vi "Find Edges.vi"(7 "Find Edge setting":T8={"Options"={"Search Direction"=0, "Edge Options"={"Edge Polarity"=0, "Kernel Size"=3, "Width"=3, "Minimum Edge Strength"=10.0, "Interpolation Type"=enum."Bilinear Fixed", "Data Processing Method"=enum."Average"}, "Show Search Area"=FALSE, "Show Search Lines"=FALSE, "Show Edges Found"=FALSE, "Show Result"=TRUE, "Search Area Color"=65280, "Search Lines Color"=255, "Edge Locations Color"=16776960, "Result Color"=16711680, "Overlay Group Name"=""}, "Line Fit Options"={"Number of Lines"=1, "Type"=enum."First Edge Rake", "Min. Score"=10.0, "Max. Score"=1000.0, "Orientation"=0.0, "Angle Range"=45.0, "Angle Tolerance"=1.0, "Step Size"=7, "Min. SNR (db)"=0.0, "Min. Points (%)"=25.0, "Hough Iterations"=5}} {"Options"."Search Direction" items=["Left to Right", "Right to Left", "Top to Bottom", "Bottom to Top"]; "Options"."Edge Options"."Edge Polarity" items=["All Edges", "Rising Edges", "Falling Edges"]; "Options"."Edge Options"."Minimum Edge Strength" format="%.2f"; "Options"."Edge Options"."Width" step=2; "Options"."Edge Options"."Kernel Size" step=2; "Line Fit Options"."Min. Points (%)" min=0.0 max=100.0; "Line Fit Options"."Min. SNR (db)" min=0.0; "Line Fit Options"."Max. Score" min=0.0 max=1024.0; "Line Fit Options"."Min. Score" min=0.0 max=1024.0 step=1.0}, 8 "error in (no error)":errorcluster, 9 "Matches (pixel)":T9, 10 "ROI Descriptor":T1 {"Contours"."Type" items=["No Selection", "Point", "Line", "Rectangle", "Oval", "Polygon", "Freehand Region", "Annulus", "Unused2", "Unused3", "Broken Line", "Freehand Line", "Rotated Rectangle"]}, 11 "Image":T3) -> (0 "error out":errorcluster, 1 "Straight Edges":T2(array[cluster]) {"Point2 (Real-World)"."Y" format="%.2f"; "Point2 (Real-World)"."X" format="%.2f"; "Point1 (Real-World)"."Y" format="%.2f"; "Point1 (Real-World)"."X" format="%.2f"; "Point2 (Pixels)"."Y" format="%.2f"; "Point2 (Pixels)"."X" format="%.2f"; "Point1 (Pixels)"."Y" format="%.2f"; "Point1 (Pixels)"."X" format="%.2f"}, 2 "Found Edge?":bool, 3 "Image Out":T3)   [LabVIEW 2017]
uses:
  <vilib>/vision/Measure.llb/Edge Options.ctl
  <vilib>/vision/Measure.llb/Edge Polarity.ctl
  <vilib>/vision/Measure.llb/Straight Edge Options.ctl
  <vilib>/vision/Measure.llb/Straight Edge Process.ctl
  <vilib>/vision/Image Controls.llb/IMAQ Image.ctl
  <vilib>/vision/NI_Vision_Development_Module.lvlib
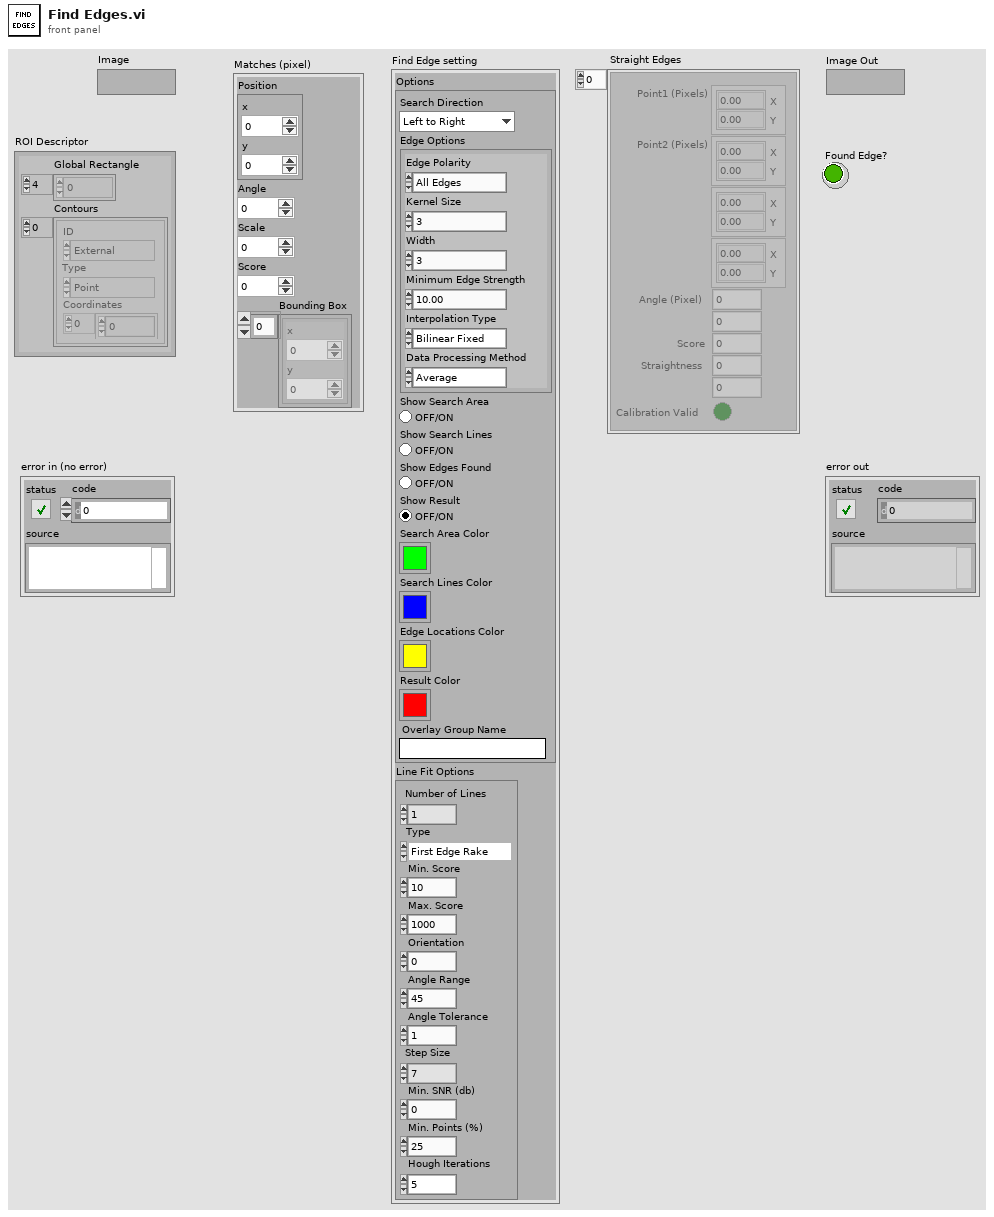
[diagram p1: front panel]
types:
  T1 = typedef "ROI Descriptor" = cluster{"Global Rectangle":i32[], "Contours":cluster{"ID":enum32{"External", "Internal"}, "Type":u32, "Coordinates":i32[]}[]}
  T2 = cluster{"Point1 (Pixels)":cluster{"X":sgl, "Y":sgl}, "Point2 (Pixels)":cluster{"X":sgl, "Y":sgl}, "Point1 (Real-World)":cluster{"X":sgl, "Y":sgl}, "Point2 (Real-World)":cluster{"X":sgl, "Y":sgl}, "Angle (Pixel)":dbl, "Angle (Real-World)":dbl, "Score":dbl, "Straightness":dbl, "Average SNR (db)":dbl, "Calibration Valid":bool}[]
  T3 = typedef "IMAQ Image.ctl" = refnum<image>
  T4 = typedef "Edge Options.ctl" = cluster{"Edge Polarity":T5, "Kernel Size":u32, "Width":u32, "Minimum Edge Strength":sgl, "Interpolation Type":enum32{"Zero Order", "Bilinear", "Quadratic", "Cubic", "Bilinear Fixed"}, "Data Processing Method":enum32{"Average", "Median"}}
  T5 = typedef "Edge Polarity.ctl" = u32
  T6 = typedef "Straight Edge Options.ctl" = cluster{"Number of Lines":i32, "Type":T7, "Min. Score":dbl, "Max. Score":dbl, "Orientation":dbl, "Angle Range":dbl, "Angle Tolerance":dbl, "Step Size":u32, "Min. SNR (db)":dbl, "Min. Points (%)":dbl, "Hough Iterations":i32}
  T7 = typedef "Straight Edge Process.ctl" = enum32{"First Edge Rake", "Best Edge Rake", "Hough Edge Rake", "First Edge Projection", "Best Edge Projection"}
  T8 = cluster{"Options":cluster{"Search Direction":u32, "Edge Options":T4, "Show Search Area":bool, "Show Search Lines":bool, "Show Edges Found":bool, "Show Result":bool, "Search Area Color":u32, "Search Lines Color":u32, "Edge Locations Color":u32, "Result Color":u32, "Overlay Group Name":string}, "Line Fit Options":T6}
  T9 = cluster{"Position":cluster{"x":sgl, "y":sgl}, "Angle":sgl, "Scale":sgl, "Score":sgl, "Bounding Box":cluster{"x":sgl, "y":sgl}[]}
  T10 = enum16{"Horizontal Motion only", "Vertical Motion only", "Horizontal and Vertical Motion", "Horizontal, Vertical and Angular"}
  T11 = cluster{"Search Direction":u32, "Edge Options":T4, "Show Search Area":bool, "Show Search Lines":bool, "Show Edges Found":bool, "Show Result":bool, "Search Area Color":u32, "Search Lines Color":u32, "Edge Locations Color":u32, "Result Color":u32, "Overlay Group Name":string}
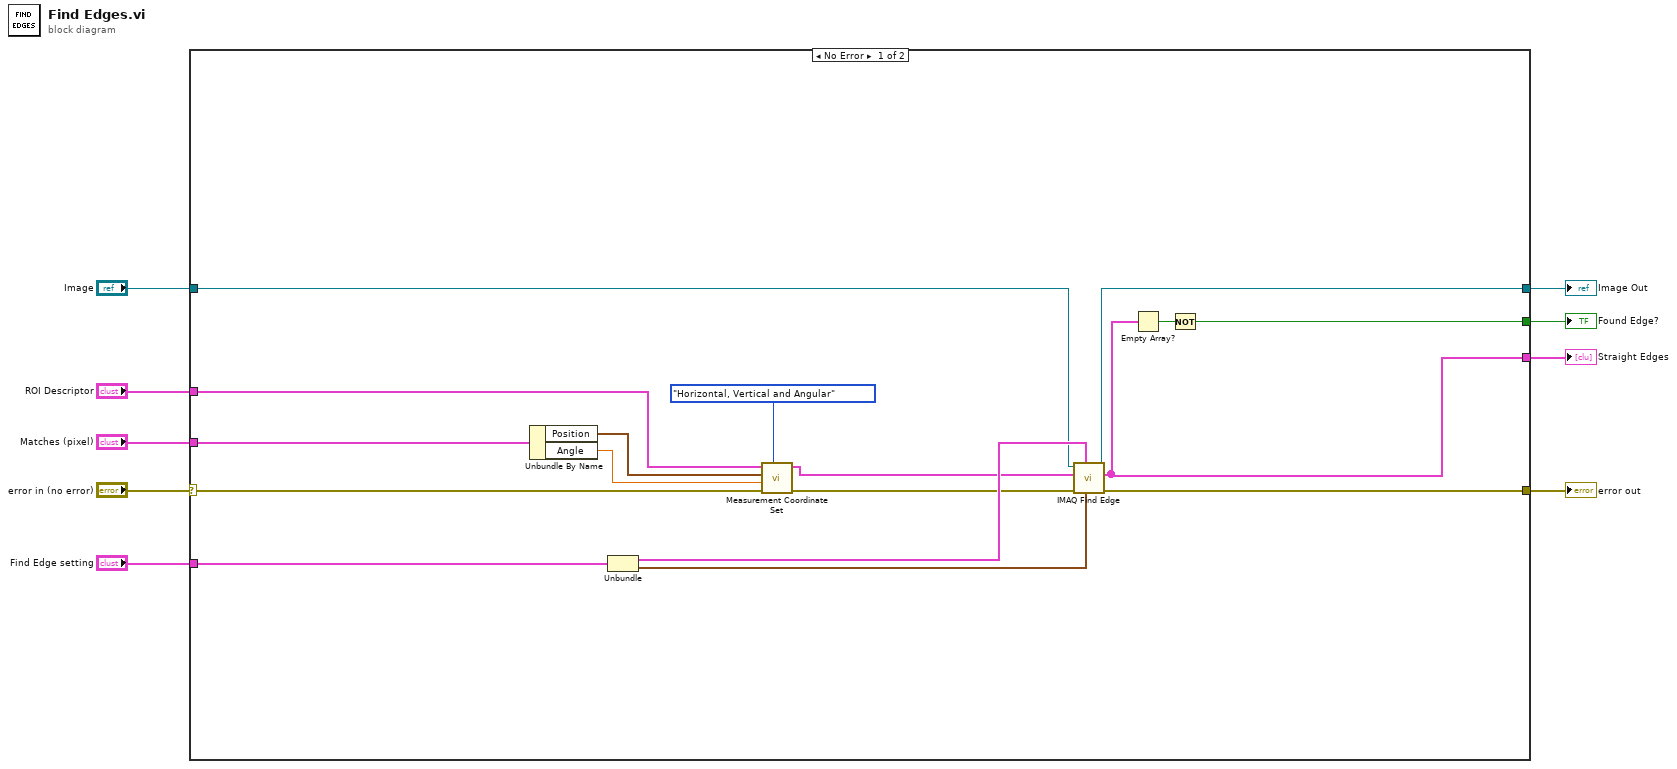
[diagram p0: block diagram]
diagram:
  n1 = case shown="No Error" "error in (no error)" {
    selector: "error in (no error)" -> [w14 w28]
    tunnel: [w24 w28] -> w8
    tunnel: "Matches (pixel)" -> [w26 _]
    tunnel: "Image" -> [w12 w27]
    tunnel: "Find Edge setting" -> [w23 _]
    tunnel: [w20 w27] -> w4
    tunnel: [w18 _] -> w3
    tunnel: [w16 _] -> w2
    tunnel: "ROI Descriptor" -> [w11 _]
    frame No Error {
      n2 = Unbundle By Name(w26) -> ("Position"=w25:cluster{"x":sgl, "y":sgl}, "Angle"=w17:sgl)
      n3 = Unbundle(w23) -> ("Options"=w22:T11, "Line Fit Options"=w21:T6)
      n4 = call "Measurement Coordinate Set.vi"("CoordSys Type"=T10."Horizontal, Vertical and Angular", "error in (no error)"=w14, "Angle (deg)"=w17, "Origin"=w25, "ROI Descriptor"=w11) -> ("error out"=w13:errorcluster, "ROI Descriptor out"=w10:T1)  [unwired: 4 in, 1 out]
      n5 = call "IMAQ Find Edge"("Line Fit Options"=w21, "Options"=w22, "error in (no error)"=w13, "ROI Descriptor"=w10, "Image"=w12) -> ("error out"=w24:errorcluster, "Straight Edges"=w16:T2, "Image Out"=w20:T3)  [unwired: 3 in, 1 out]
      n6 = Empty Array?(array=w16) -> (empty?=w19:bool)
      n7 = Not(x=w19) -> (.not. x?=w18:bool)
    }
    frame Error {
    }
  }
  "error out" <- w8
  "Image Out" <- w4
  "Found Edge?" <- w3
  "Straight Edges" <- w2
